vi "RSZVB Write Calibration Data.vi"(5 "Port 1 (1)":i32=1, 6 "Calibration Data":dbl[](array[numeric]) format="%^.3e", 7 "Port 2 (1)":i32=1, 8 "error in (no error)":errorcluster {"code" format="%.0x"}, 9 "Error Term Parameters (0: Directivity)":i32(ring) items=["Directivity", "Source Match", "Reflection Tracking", "Isolation", "Load Match", "Transmission Tracking", "G11", "G12", "G21", "G22", "H11", "H12", "H21", "H22"], 10 "Channel (1)":i32=1, 11 "VISA session":refnum<visa-resource-name>) -> (0 "error out":errorcluster {"code" format="%.0x"}, 3 "dup VISA session":refnum<visa-resource-name>)   [LabVIEW 2011]
doc: "This VI writes system error correction data for a specific channel, calibration method, and port combination <Port 1>, <Port 2>.\n\nRemote-control command(s):\nFORMat ASCII\nFORMat REAL,32\nSYSTem:COMMunicate:GPIB:SELF:RTERminator EOI\n[SENSe<Ch>:]CORRection:CDATa"
uses:
  _utility/RSZVB Global Data.vi
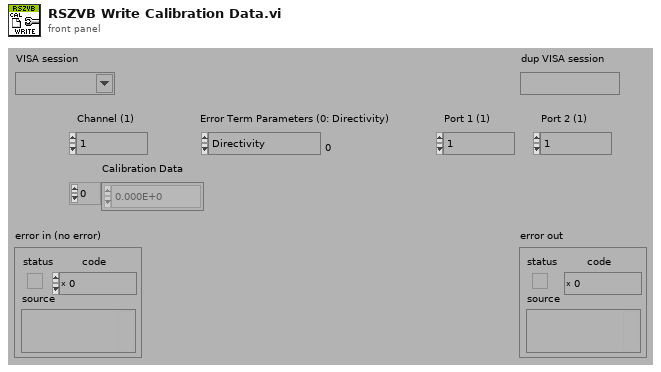
[diagram p1: front panel]
types:
  T1 = cluster{"Error Checking (T: On)":bool, "Installed Options":string[], "Data Valid?":bool, "Ports":i32, "Model":string[], "Option Checking (T: On)":bool}[]
  T2 = cluster{"Error Checking (T: On)":bool, "Installed Options":string[], "Data Valid?":bool, "Ports":i32, "Model":string[], "Option Checking (T: On)":bool}
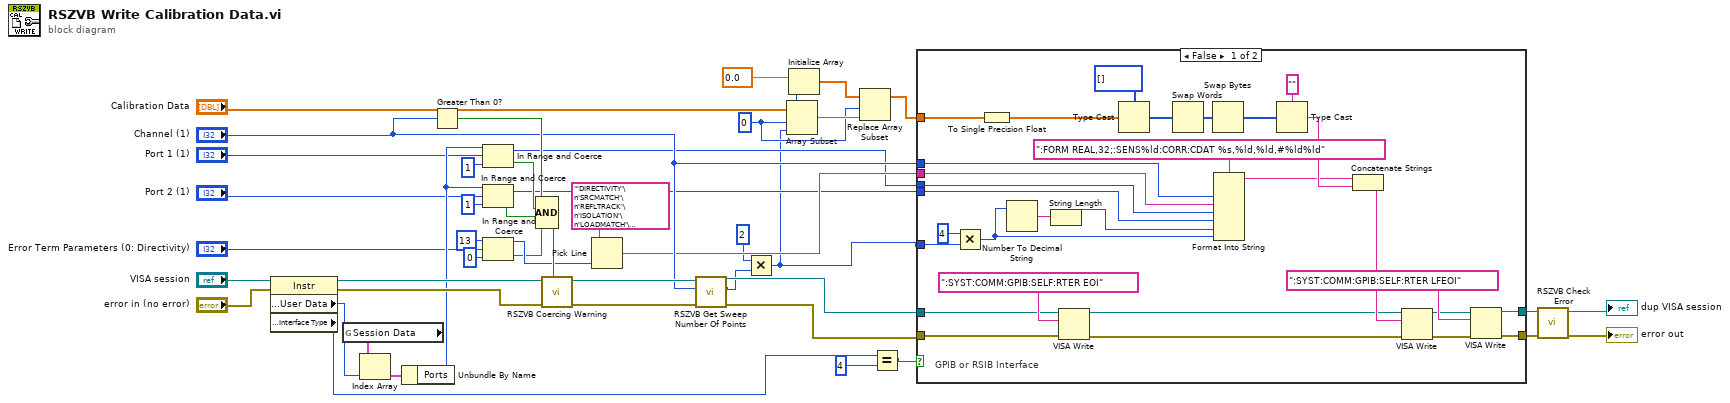
[diagram p0: block diagram]
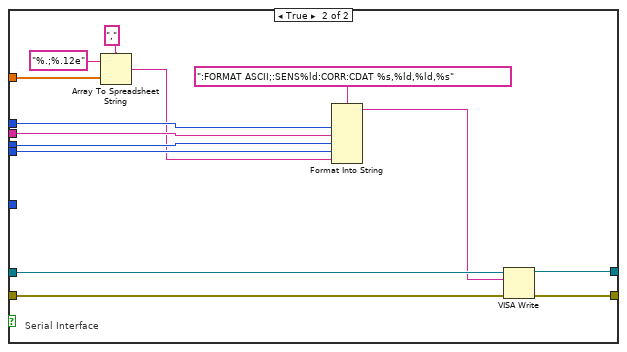
[diagram p2: hidden frame]
diagram:
  w18 = 0 ("index")
  n1 = property class="Instr"(reference="VISA session", error in="error in (no error)") -> (reference out=w39:refnum<visa-resource-name>, error out=w40:errorcluster, "General Settings:User Data"=w41:u32, "Interface Information:Interface Type"=w16:u16)
  n2 = global read "RSZVB Global Data.vi" "Session Data"() -> (w42:T1)
  n3 = Index Array(array=w42, index=w41) -> (element=w43:T2)
  n4 = Unbundle By Name(w43) -> ("Ports"=w30:i32)
  n5 = Greater Than 0?(x="Channel (1)") -> (x > 0?=w44:bool)
  n6 = In Range and Coerce(upper limit=w30, x="Port 1 (1)", lower limit=1) -> (coerced(x)=w13:i32, In Range?=w33:bool)
  n7 = In Range and Coerce(upper limit=w30, x="Port 2 (1)", lower limit=1) -> (coerced(x)=w12:i32, In Range?=w32:bool)
  n8 = In Range and Coerce(upper limit=13 ("lower limit"), x="Error Term Parameters (0: Directivity)", lower limit=0) -> (coerced(x)=w35:i32, In Range?=w31:bool)
  n9 = Compound Arithmetic op=AND(w44, w33, w32, w31) -> (w45:bool)
  n10 = call "RSZVB Coercing Warning.vi"("In Range?"=w45, "error in (no error)"=w40, "VISA session"=w39) -> ("error out"=w24:errorcluster, "dup VISA session"=w23:refnum<visa-resource-name>)  [unwired: 7 in]
  n11 = Pick Line(multi-line string="'DIRECTIVITY'\n'SRCMATCH'\n'REFLTRACK'\n'ISOLATION'\n'LOADMATCH'\n'TRANSTRACK'\n'G11'\n'G12'\n'G21'\n'G22'\n'H11'\n'H12'\n'H21'\n'H22'", line index=w35) -> (output string=w14:string)  [unwired: 1 in]
  n12 = call "RSZVB Get Sweep Number Of Points.vi"("error in (no error)"=w24, "Channel (1)"="Channel (1)", "VISA session"=w23) -> ("error out"=w11:errorcluster, "Number Of Points"=w2:i32, "dup VISA session"=w10:refnum<visa-resource-name>)  [unwired: 6 in]
  n13 = Multiply(x=2, y=w2) -> (x*y=w3:i32)
  n14 = Array Subset(array="Calibration Data", index=w18, length=w3) -> (w20:dbl[])
  n15 = Initialize Array(0.0 ("element"), w3) -> (w19:dbl[])
  n16 = Replace Array Subset(array=w19, new element=w20, index=w18) -> (w17:dbl[])
  n17 = Equal?(x=w16, y=u16 4) -> (x = y?=w9:bool)
  n18 = case shown="False" w9 {
    tunnel: [w74 w89] -> w6
    tunnel: [w73 w90] -> w7
    tunnel: w17 -> [w54 w83]
    tunnel: w11 -> [w64 w87]
    tunnel: w10 -> [w63 w88]
    tunnel: "Channel (1)" -> [w55 w81]
    tunnel: w3 -> [w52 _]
    tunnel: w14 -> [w51 w80]
    tunnel: w13 -> [w49 w79]
    tunnel: w12 -> [w50 w78]
    frame False {
      # "GPIB or RSIB Interface"
      n19 = Multiply(x=u32 4, y=w52) -> (x*y=w47:u32)
      n20 = To Single Precision Float(number=w54) -> (single precision float=w53:sgl[])
      n21 = Number To Decimal String(number=w47) -> (decimal integer string=w59:string)  [unwired: 1 in]
      n22 = String Length(string=w59) -> (length=w48:i32)
      n23 = VISA Write(VISA resource name=w63, write buffer=":SYST:COMM:GPIB:SELF:RTER EOI", error in (no error)=w64) -> (VISA resource name out=w68:refnum<visa-resource-name>, error out=w65:errorcluster)  [unwired: 1 out]
      n24 = Type Cast(type=i32[] [], x=w53) -> (*(type *) &x=w75:i32[])
      n25 = Swap Words(1:w75) -> (0:w58:i32[])
      n26 = Swap Bytes(anything=w58) -> (byte swapped=w76:i32[])
      n27 = Format Into String(format string=":FORM REAL,32;:SENS%ld:CORR:CDAT %s,%ld,%ld,#%ld%ld", w55, w51, w49, w50, w48, w47) -> (resulting string=w60:string)  [unwired: 2 in, 1 out]
      n28 = Type Cast(type="", x=w76) -> (*(type *) &x=w61:string)
      n29 = Concatenate Strings(w60, w61) -> (w72:string)
      n30 = VISA Write(VISA resource name=w68, write buffer=w72, error in (no error)=w65) -> (VISA resource name out=w67:refnum<visa-resource-name>, error out=w66:errorcluster)  [unwired: 1 out]
      n31 = VISA Write(VISA resource name=w67, write buffer=":SYST:COMM:GPIB:SELF:RTER LFEOI", error in (no error)=w66) -> (VISA resource name out=w73:refnum<visa-resource-name>, error out=w74:errorcluster)  [unwired: 1 out]
    }
    frame True {
      # "Serial Interface"
      n32 = Array To Spreadsheet String(delimiter (Tab)=",", array=w83, 3:"%.;%.12e" ("format string")) -> (spreadsheet string=w77:string)
      n33 = Format Into String(format string=":FORMAT ASCII;:SENS%ld:CORR:CDAT %s,%ld,%ld,%s", w81, w80, w79, w78, w77) -> (resulting string=w82:string)  [unwired: 2 in, 1 out]
      n34 = VISA Write(VISA resource name=w88, write buffer=w82, error in (no error)=w87) -> (VISA resource name out=w90:refnum<visa-resource-name>, error out=w89:errorcluster)  [unwired: 1 out]
    }
  }
  n35 = call "RSZVB Check Error.vi"("error in (no error)"=w6, "VISA session"=w7) -> ("error out"=→"error out":errorcluster, "dup VISA session"=→"dup VISA session":refnum<visa-resource-name>)  [unwired: 8 in]
